vi "measureEchoes_timeLapse.vi"(3 "Read freqs. \nfrom textfile":bool, 5 "Cluster":T2={"span"=600000000.0, "rbw"=1000.0, "enableVBW"=FALSE, "vbw"=0.0, "traceLength"=64001, "window"=0, "verticalUnit"=0, "center freq"=300000000.0} {"verticalUnit" items=["SpectrumVerticalUnit_dBm", "SpectrumVerticalUnit_Watt", "SpectrumVerticalUnit_Volt", "SpectrumVerticalUnit_Amp", "SpectrumVerticalUnit_dBmV"]; "window" items=["SpectrumWindow_Kaiser", "SpectrumWindow_Mil6dB", "SpectrumWindow_BlackmanHarris", "SpectrumWindow_Rectangle", "SpectrumWindow_FlatTop", "SpectrumWindow_Hann"]; "traceLength" items=["801"=801, "2401"=2401, "4001"=4001, "8001"=8001, "10401"=10401, "16001"=16001, "32001"=32001, "64001"=64001]}, 6 "error in":errorcluster, 7 "Echo measurement time":i32=30, 8 "Burn time/OFC measurement time":i32=30, 9 "Folder for all data (Don't forget the last slash!)":string) -> (0 "error out":errorcluster)   [LabVIEW 2016]
uses:
  <vilib>/Utility/file.llb/Read Delimited Spreadsheet (DBL).vi
  <vilib>/Utility/file.llb/Write Delimited Spreadsheet (DBL).vi
panel:
  in  "Serial Configuration":T1={"Baud Rate"=9600, "Parity"=0, "Data Bits"=8, "Flow Control"=4} {"Baud Rate" items=["300"=300, "600"=600, "1200"=1200, "2400"=2400, "4800"=4800, "9600"=9600, "19200"=19200]; "Parity" items=["None", "Odd", "Even", "Mark", "Space"]; "Data Bits" items=["7"=7, "8"=8]; "Flow Control" items=["None", "XON/XOFF", "RTS/CTS", "XON/XOFF & RTS/CTS", "DTR/DSR", "XON/XOFF & DTR/DSR"]}
  in  "Agilent 33250A address":refnum<visa-resource-name>="GPIB0::4::INSTR"
  out "Last saved trace":sgl[](graph)
  in  "stop":bool
  out "RSA error out":errorcluster
  out "Real-time trace":sgl[](graph)
  out "Current set #":i32
  out "Current freq.":dbl
  in  "freqs. file":path
  in  "Shuffle?":bool
  in  "Start freq":dbl=100000.0 format="%0.2e"
  in  "End freq":dbl=20000000.0 format="%0.2e"
  in  "Freq step":i32=100000 format="%.2e"
  in  "Mod shape":enum16{"Triangle", "Sine"}(ring)
  # "RSA settings"
  # "Suppose you want to collect comb data, first ascending, then descending.\n\nIn Matlab, create a 1xM array \ncontaining all modulation freqs (Hz) in the ascending sequence; then create a 1xN array for the descending case. Note that M != N is fine.\n\nfid= fopen(FILENAME, 'w');\nfprintf(fid,'%d\\t', ARRAY1);\nfprintf(fid,'\\r\\n');\nfprintf(fid,'%d\\t',ARRAY2);\n... \n(for more sets, repeat as needed)\nfclose(fid);\n\nNow find the file you just made:"
  # "Modulation settings"
  # "(zero-indexed)"
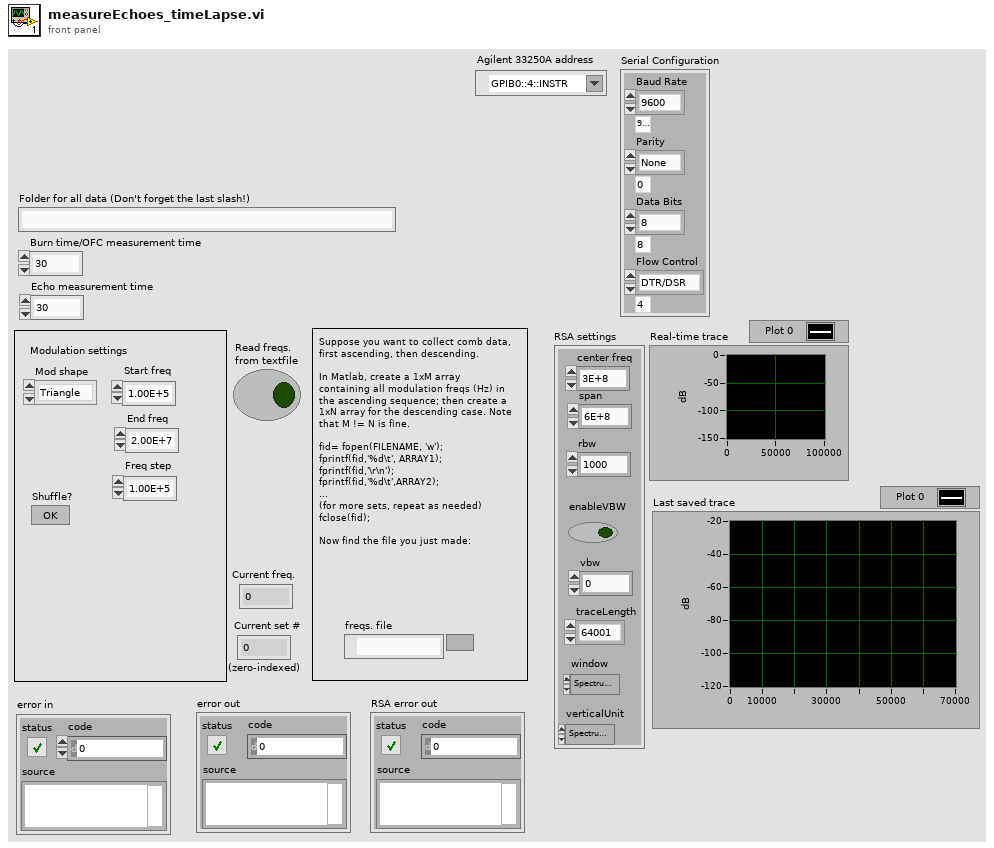
[diagram p1: front panel]
types:
  T1 = cluster{"Baud Rate":u32, "Parity":u16, "Data Bits":u16, "Flow Control":u16}
  T2 = cluster{"span":dbl, "rbw":dbl, "enableVBW":bool, "vbw":dbl, "traceLength":u16, "window":u32, "verticalUnit":u32, "center freq":dbl}
  T3 = cluster{"span":dbl, "rbw":dbl, "enableVBW":bool, "vbw":dbl, "traceLength":u16, "window":u32, "verticalUnit":u32}
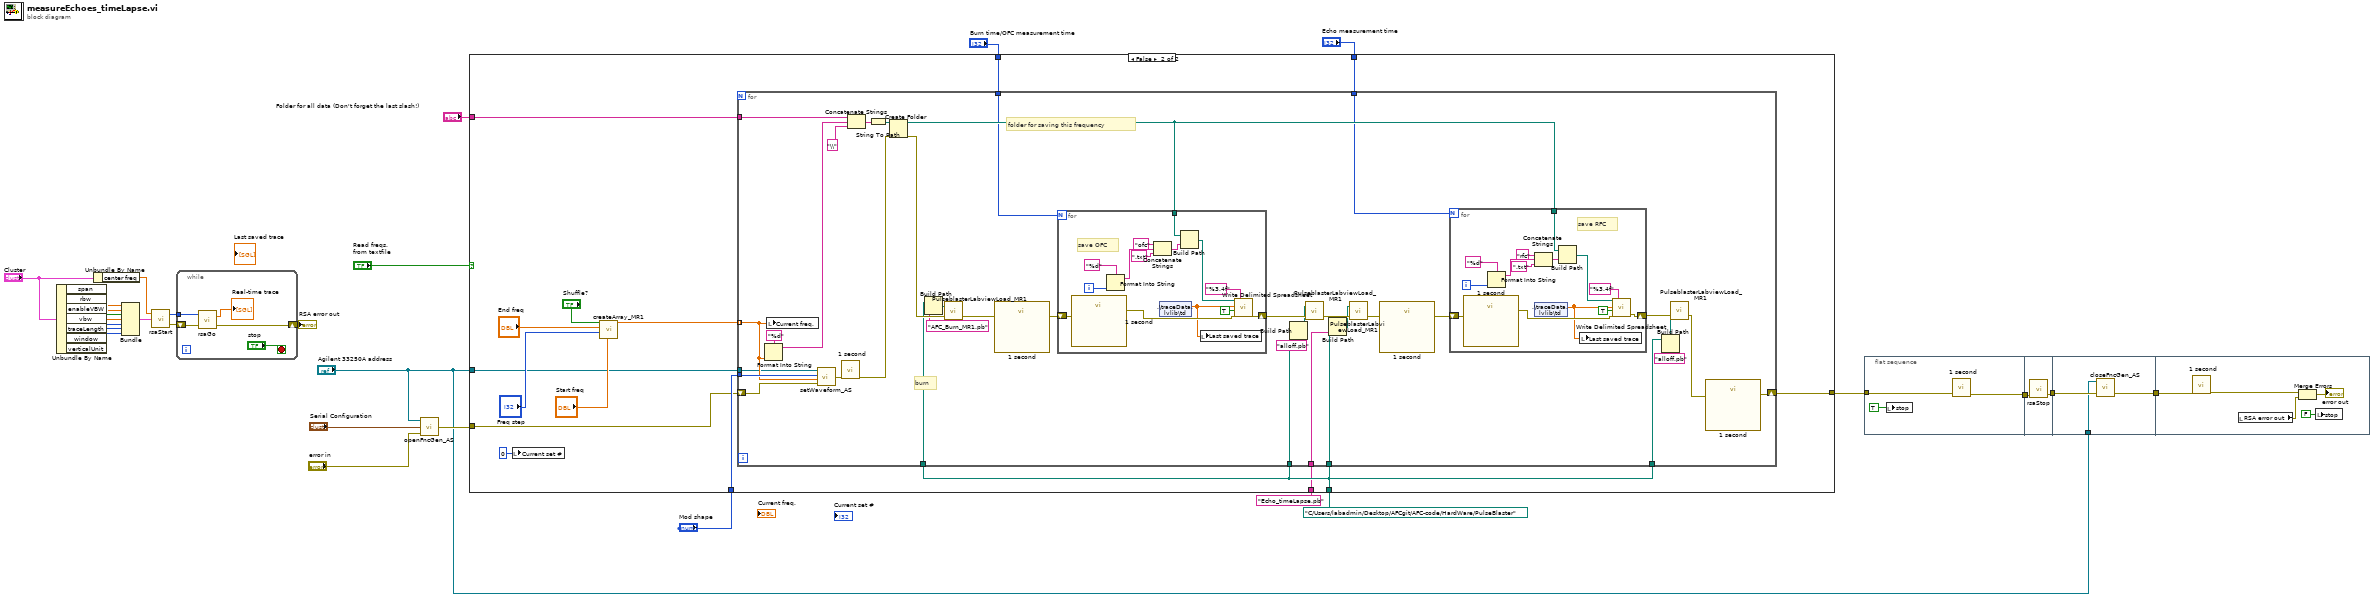
[diagram p0: block diagram]
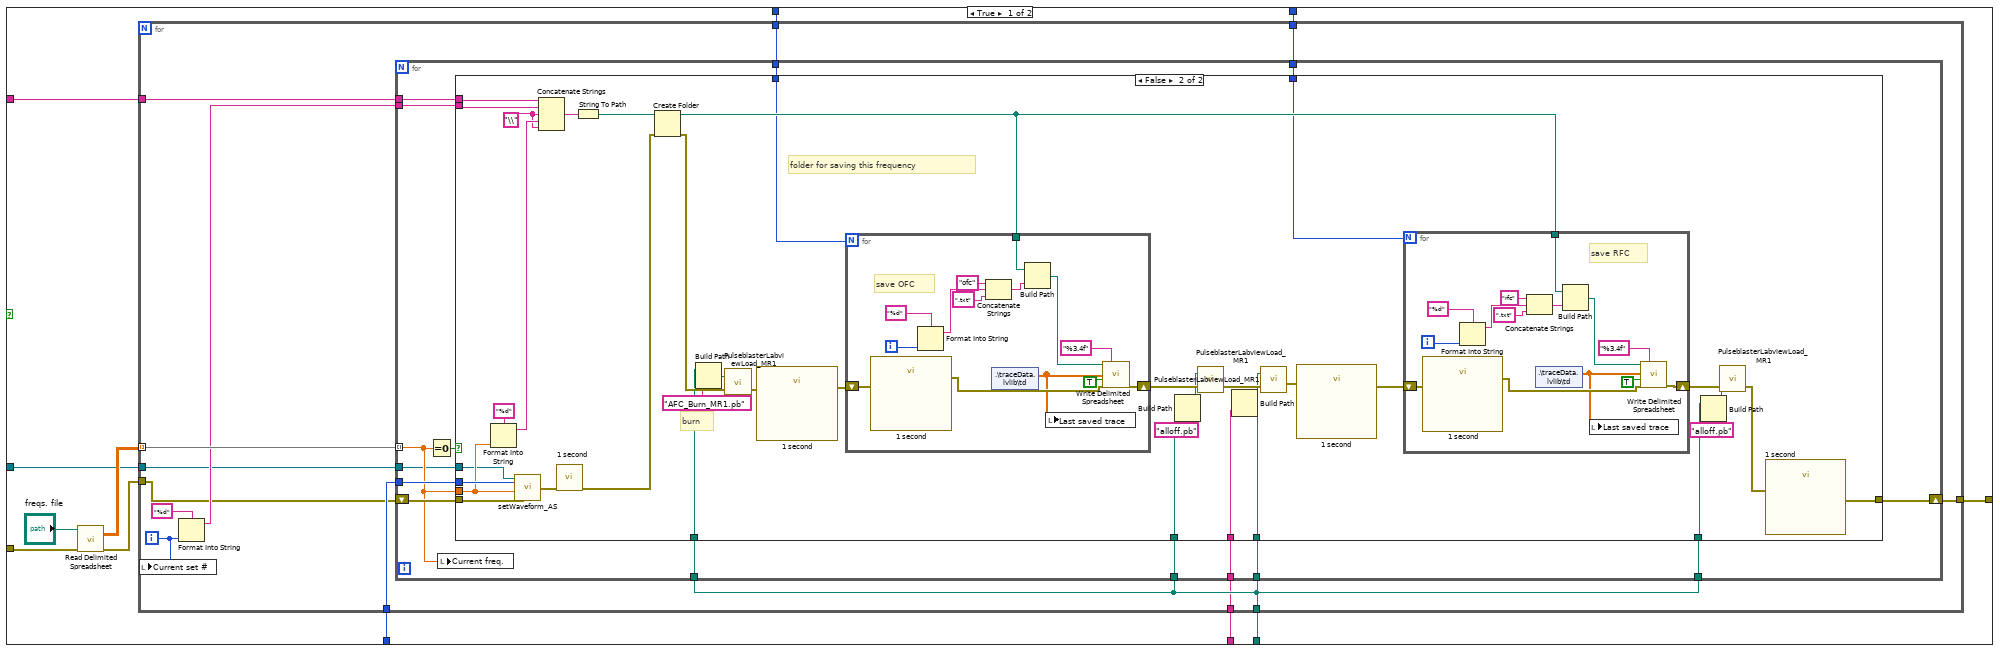
[diagram p2: hidden frame]
diagram:
  n1 = Unbundle By Name("Cluster") -> ("span"=w21:dbl, "rbw"=w22:dbl, "enableVBW"=w23:bool, "vbw"=w24:dbl, "traceLength"=w25:u16, "window"=w26:u32, "verticalUnit"=w27:u32)
  n2 = Unbundle By Name("Cluster") -> ("center freq"=w15:dbl)
  n3 = Bundle("span"=w21, "rbw"=w22, "enableVBW"=w23, "vbw"=w24, "traceLength"=w25, "window"=w26, "verticalUnit"=w27) -> (w14:T3)  [unwired: 1 in]
  n4 = call "rsaStart.vi"("Cluster"=w14, "center freq"=w15) -> ("error out"=w12:errorcluster, "traceLength"=w13:u16)  [unwired: 1 in]
  n5 = while {
    tunnel: w13 -> [w33]
    shift-right: [w31] -> w11
    shift-left: w12 -> [w30]
    stop <- "stop" stop-if-true
    n6 = call "rsaGo.vi"("error in"=w30, "Trace length"=w33) -> ("error out"=w31:errorcluster, "traceData out"=→"Real-time trace":sgl[])  [unwired: 1 in]
  }
  "RSA error out" <- w11
  n7 = call "openFncGen_AS.vi"("error in (no error)"="error in", "Serial Configuration"="Serial Configuration", "VISA resource name"="Agilent 33250A address") -> ("error out"=w6:errorcluster)
  n8 = case shown="False" "Read freqs. \nfrom textfile" {
    tunnel: "Folder for all data (Don't forget the last slash!)" -> [w45 w155]
    tunnel: path "C:/Users/labadmin/Desktop/AFCgit/AFC-code/HardWare/PulseBlaster" ("base path") -> [w37 w154]
    tunnel: "Burn time/OFC measurement time" -> [w44 w153]
    tunnel: "Echo measurement time" -> [w43 w152]
    tunnel: w6 -> [w41 w143]
    tunnel: "Mod shape" -> [w38 w146]
    tunnel: [w36 w144] -> w28
    tunnel: "Echo_timeLapse.pb" ("name or relative path") -> [w35 w142]
    tunnel: "Agilent 33250A address" -> [w34 w141]
    frame True {
      n9 = call-poly <vilib>:"Read Delimited Spreadsheet.vi"("file path (dialog if empty)"="freqs. file", "error in (no error)"=w41) -> ("all rows"=w40:dbl[][], "error out"=w39:errorcluster)  [unwired: 8 in, 4 out]
      n10 = for {
        tunnel: [w58] -> w36
        tunnel: w45 -> [w57]
        tunnel: w37 -> [w56]
        tunnel: w44 -> [w55]
        tunnel: w43 -> [w54]
        tunnel: w40 -> [w53] mode=indexing
        tunnel: w39 -> [w48]
        tunnel: w38 -> [w50]
        tunnel: w35 -> [w47]
        tunnel: w34 -> [w46]
        i -> [w49]
        n11 = local write "Current set #"(w49) -> ()
        n12 = Format Into String(format string="%d", w49) -> (resulting string=w51:string)  [unwired: 2 in, 1 out]
        n13 = for {
          tunnel: w53 -> [w61] mode=indexing
          tunnel: w50 -> [w73]
          shift-right: [w72] -> w58
          shift-left: w48 -> [w71]
          tunnel: w57 -> [w63]
          tunnel: w56 -> [w70]
          tunnel: w56 -> [w69]
          tunnel: w56 -> [w68]
          tunnel: w56 -> [w67]
          tunnel: w55 -> [w66]
          tunnel: w54 -> [w65]
          tunnel: w51 -> [w64]
          tunnel: w47 -> [w60]
          tunnel: w46 -> [w59]
          n14 = Equal To 0?(x=w61) -> (x = 0?=w62:bool)
          n15 = local write "Current freq."(w61) -> ()
          n16 = case shown="False" w62 {
            tunnel: w73 -> [_ w78]
            tunnel: [w74 w81] -> w72
            tunnel: w71 -> [w74 w76]
            tunnel: w70 -> [_ w104]
            tunnel: w69 -> [_ w101]
            tunnel: w68 -> [_ w99]
            tunnel: w67 -> [_ w96]
            tunnel: w66 -> [_ w94]
            tunnel: w65 -> [_ w93]
            tunnel: w64 -> [_ w88]
            tunnel: w63 -> [_ w89]
            tunnel: w61 -> [_ w77]
            tunnel: w60 -> [_ w80]
            tunnel: w59 -> [_ w75]
            frame True {
            }
            frame False {
              w91 = "\\" ("string")
              # "folder for saving this frequency"
              # "burn"
              n17 = Format Into String(format string="%d", w77) -> (resulting string=w92:string)  [unwired: 2 in, 1 out]
              n18 = call "setWaveform_AS.vi"("error in (no error)"=w76, "Frequency (1000 Hz)"=w77, "Enum"=w78, "VISA resource name"=w75) -> ("error out"=w79:errorcluster)
              n19 = Concatenate Strings(w89, w88, w91, w92, w91) -> (w87:string)
              n20 = call "1 second"("error in (no error)"=w79) -> ("error out"=w108:errorcluster)  [unwired: 10 in]
              n21 = String To Path(string=w87) -> (path=w105:path)
              n22 = Create Folder(path (use dialog)=w105, error in=w108) -> (created path=w106:path, error out=w107:errorcluster)  [unwired: 1 in, 1 out]
              n23 = Build Path(base path=w104, name or relative path="AFC_Burn_MR1.pb") -> (appended path=w102:path)
              n24 = call "PulseblasterLabviewLoad_MR1.vi"("error in (no error)"=w107, "Input file"=w102) -> ("error out"=w86:errorcluster)  [unwired: 1 out]
              n25 = call "1 second"("error in (no error)"=w86) -> ("error out"=w85:errorcluster)  [unwired: 10 in]
              n26 = for {
                N: w94 -> [_]
                shift-right: [w139] -> w109
                shift-left: w85 -> [w129]
                tunnel: w106 -> [w132]
                i -> [w130]
                # "save OFC"
                n27 = call "1 second"("error in (no error)"=w129) -> ("error out"=w128:errorcluster)  [unwired: 10 in]
                n28 = Format Into String(format string="%d", w130) -> (resulting string=w135:string)  [unwired: 2 in, 1 out]
                n29 = Concatenate Strings("ofc" ("string"), w135, ".txt" ("string")) -> (w134:string)
                n30 = shared-variable ".\\traceData.lvlib\\td"() -> (w127:dbl[])  [unwired: 1 in, 1 out]
                n31 = Build Path(base path=w132, name or relative path=w134) -> (appended path=w138:path)
                n32 = local write "Last saved trace"(w127) -> ()
                n33 = call-poly <vilib>:"Write Delimited Spreadsheet.vi"("file path (dialog if empty)"=w138, "format (%.3f)"="%3.4f", "1D data"=w127, "append to file? (new file:F)"=TRUE, "error in (no error)"=w128) -> ("error out"=w139:errorcluster)  [unwired: 9 in, 1 out]
              }
              n34 = Build Path(base path=w99, name or relative path="alloff.pb") -> (appended path=w98:path)
              n35 = call "PulseblasterLabviewLoad_MR1.vi"("error in (no error)"=w109, "Input file"=w98) -> ("error out"=w110:errorcluster)  [unwired: 1 out]
              n36 = Build Path(base path=w101, name or relative path=w80) -> (appended path=w100:path)
              n37 = call "PulseblasterLabviewLoad_MR1.vi"("error in (no error)"=w110, "Input file"=w100) -> ("error out"=w84:errorcluster)  [unwired: 1 out]
              n38 = call "1 second"("error in (no error)"=w84) -> ("error out"=w83:errorcluster)  [unwired: 10 in]
              n39 = for {
                N: w93 -> [_]
                shift-right: [w125] -> w111
                shift-left: w83 -> [w115]
                tunnel: w106 -> [w117]
                i -> [w121]
                # "save RFC"
                n40 = call "1 second"("error in (no error)"=w115) -> ("error out"=w114:errorcluster)  [unwired: 10 in]
                n41 = Format Into String(format string="%d", w121) -> (resulting string=w120:string)  [unwired: 2 in, 1 out]
                n42 = Concatenate Strings("rfc" ("string"), w120, ".txt" ("string")) -> (w119:string)
                n43 = shared-variable ".\\traceData.lvlib\\td"() -> (w113:dbl[])  [unwired: 1 in, 1 out]
                n44 = Build Path(base path=w117, name or relative path=w119) -> (appended path=w124:path)
                n45 = local write "Last saved trace"(w113) -> ()
                n46 = call-poly <vilib>:"Write Delimited Spreadsheet.vi"("file path (dialog if empty)"=w124, "format (%.3f)"="%3.4f", "1D data"=w113, "append to file? (new file:F)"=TRUE, "error in (no error)"=w114) -> ("error out"=w125:errorcluster)  [unwired: 9 in, 1 out]
              }
              n47 = Build Path(base path=w96, name or relative path="alloff.pb") -> (appended path=w95:path)
              n48 = call "PulseblasterLabviewLoad_MR1.vi"("error in (no error)"=w111, "Input file"=w95) -> ("error out"=w82:errorcluster)  [unwired: 1 out]
              n49 = call "1 second"("error in (no error)"=w82) -> ("error out"=w81:errorcluster)  [unwired: 10 in]
            }
          }
        }
      }
    }
    frame False {
      n50 = local write "Current set #"(0 ("Current set #")) -> ()
      n51 = call "createArray_MR1.vi"("Start freq"="Start freq", "Freq step"="Freq step", "End freq"="End freq", "Shuffle?"="Shuffle?") -> ("Riffled {X}"=w147:dbl[])  [unwired: 7 in]
      n52 = for {
        tunnel: w147 -> [w158] mode=indexing
        tunnel: w146 -> [w160]
        shift-right: [w164] -> w144
        shift-left: w143 -> [w159]
        tunnel: w155 -> [w171]
        tunnel: w154 -> [w181]
        tunnel: w154 -> [w178]
        tunnel: w154 -> [w176]
        tunnel: w154 -> [w173]
        tunnel: w153 -> [w170]
        tunnel: w152 -> [w169]
        tunnel: w142 -> [w161]
        tunnel: w141 -> [w157]
        # "folder for saving this frequency"
        # "burn"
        n53 = Format Into String(format string="%d", w158) -> (resulting string=w191:string)  [unwired: 2 in, 1 out]
        n54 = local write "Current freq."(w158) -> ()
        n55 = call "setWaveform_AS.vi"("error in (no error)"=w159, "Frequency (1000 Hz)"=w158, "Enum"=w160, "VISA resource name"=w157) -> ("error out"=w156:errorcluster)
        n56 = call "1 second"("error in (no error)"=w156) -> ("error out"=w186:errorcluster)  [unwired: 10 in]
        n57 = Concatenate Strings(w171, w191, "\\" ("string")) -> (w183:string)
        n58 = String To Path(string=w183) -> (path=w182:path)
        n59 = Create Folder(path (use dialog)=w182, error in=w186) -> (created path=w184:path, error out=w185:errorcluster)  [unwired: 1 in, 1 out]
        n60 = Build Path(base path=w181, name or relative path="AFC_Burn_MR1.pb") -> (appended path=w179:path)
        n61 = call "PulseblasterLabviewLoad_MR1.vi"("error in (no error)"=w185, "Input file"=w179) -> ("error out"=w166:errorcluster)  [unwired: 1 out]
        n62 = call "1 second"("error in (no error)"=w166) -> ("error out"=w167:errorcluster)  [unwired: 10 in]
        n63 = for {
          N: w170 -> [_]
          shift-right: [w219] -> w187
          shift-left: w167 -> [w209]
          tunnel: w184 -> [w212]
          i -> [w210]
          # "save OFC"
          n64 = call "1 second"("error in (no error)"=w209) -> ("error out"=w208:errorcluster)  [unwired: 10 in]
          n65 = Format Into String(format string="%d", w210) -> (resulting string=w215:string)  [unwired: 2 in, 1 out]
          n66 = Concatenate Strings("ofc" ("string"), w215, ".txt" ("string")) -> (w214:string)
          n67 = shared-variable ".\\traceData.lvlib\\td"() -> (w207:dbl[])  [unwired: 1 in, 1 out]
          n68 = Build Path(base path=w212, name or relative path=w214) -> (appended path=w218:path)
          n69 = local write "Last saved trace"(w207) -> ()
          n70 = call-poly <vilib>:"Write Delimited Spreadsheet.vi"("file path (dialog if empty)"=w218, "format (%.3f)"="%3.4f", "1D data"=w207, "append to file? (new file:F)"=TRUE, "error in (no error)"=w208) -> ("error out"=w219:errorcluster)  [unwired: 9 in, 1 out]
        }
        n71 = Build Path(base path=w176, name or relative path="alloff.pb") -> (appended path=w175:path)
        n72 = call "PulseblasterLabviewLoad_MR1.vi"("error in (no error)"=w187, "Input file"=w175) -> ("error out"=w188:errorcluster)  [unwired: 1 out]
        n73 = Build Path(base path=w178, name or relative path=w161) -> (appended path=w177:path)
        n74 = call "PulseblasterLabviewLoad_MR1.vi"("error in (no error)"=w188, "Input file"=w177) -> ("error out"=w162:errorcluster)  [unwired: 1 out]
        n75 = call "1 second"("error in (no error)"=w162) -> ("error out"=w163:errorcluster)  [unwired: 10 in]
        n76 = for {
          N: w169 -> [_]
          shift-right: [w205] -> w189
          shift-left: w163 -> [w195]
          tunnel: w184 -> [w197]
          i -> [w201]
          # "save RFC"
          n77 = call "1 second"("error in (no error)"=w195) -> ("error out"=w194:errorcluster)  [unwired: 10 in]
          n78 = Format Into String(format string="%d", w201) -> (resulting string=w200:string)  [unwired: 2 in, 1 out]
          n79 = Concatenate Strings("rfc" ("string"), w200, ".txt" ("string")) -> (w199:string)
          n80 = shared-variable ".\\traceData.lvlib\\td"() -> (w193:dbl[])  [unwired: 1 in, 1 out]
          n81 = Build Path(base path=w197, name or relative path=w199) -> (appended path=w204:path)
          n82 = local write "Last saved trace"(w193) -> ()
          n83 = call-poly <vilib>:"Write Delimited Spreadsheet.vi"("file path (dialog if empty)"=w204, "format (%.3f)"="%3.4f", "1D data"=w193, "append to file? (new file:F)"=TRUE, "error in (no error)"=w194) -> ("error out"=w205:errorcluster)  [unwired: 9 in, 1 out]
        }
        n84 = Build Path(base path=w173, name or relative path="alloff.pb") -> (appended path=w172:path)
        n85 = call "PulseblasterLabviewLoad_MR1.vi"("error in (no error)"=w189, "Input file"=w172) -> ("error out"=w165:errorcluster)  [unwired: 1 out]
        n86 = call "1 second"("error in (no error)"=w165) -> ("error out"=w164:errorcluster)  [unwired: 10 in]
      }
    }
  }
  n87 = flat-sequence {
    tunnel: w28 -> [w222]
    tunnel: [w221] -> w10
    tunnel: w10 -> [w225]
    tunnel: [w224] -> w4
    tunnel: w4 -> [w228]
    tunnel: [w227] -> w3
    tunnel: "Agilent 33250A address" -> [w226]
    tunnel: w3 -> [w230]
    frame #0 {
      n88 = local write "stop"(TRUE ("Stop")) -> ()
      n89 = call "1 second"("error in (no error)"=w222) -> ("error out"=w221:errorcluster)  [unwired: 10 in]
    }
    frame #1 {
      n90 = call "rsaStop.vi"("error in (no error)"=w225) -> ("error out"=w224:errorcluster)  [unwired: 3 in]
    }
    frame #2 {
      n91 = call "closeFncGen_AS.vi"("error in (no error)"=w228, "VISA resource name"=w226) -> ("error out"=w227:errorcluster)  [unwired: 1 in]
    }
    frame #3 {
      n92 = call "1 second"("error in (no error)"=w230) -> ("error out"=w229:errorcluster)  [unwired: 10 in]
      n93 = local read "RSA error out"() -> (w233:errorcluster)
      n94 = Merge Errors(w229, w233) -> (→"error out":errorcluster)
      n95 = local write "stop"(FALSE ("stop")) -> ()
    }
  }
